vi "disableMenueItem.vi"(3 "error in":errorcluster, 4 "ItemTag":string, 5 "All Devices (h)":string[](array[string]), 6 "MenuRef":refnum<k9>) -> (0 "error out":errorcluster, 1 "this is a Device(tag)":bool, 2 "menu reference out":refnum<k9>)   [LabVIEW 2013]
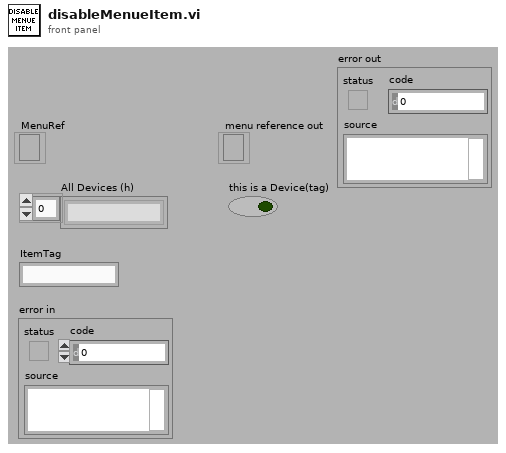
[diagram p1: front panel]
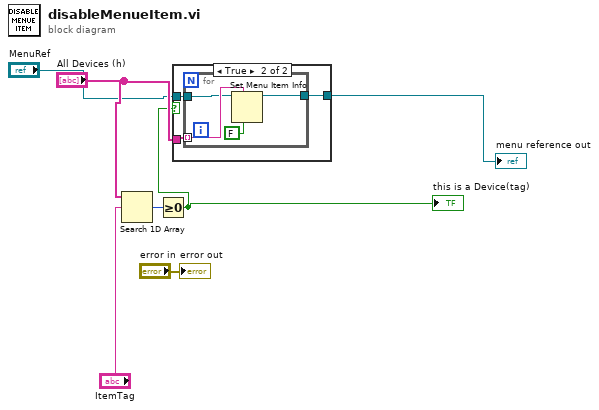
[diagram p0: block diagram]
diagram:
  n1 = Search 1D Array(1D array="All Devices (h)", element="ItemTag") -> (index of element=w3:i32)  [unwired: 1 in]
  n2 = Greater Or Equal To 0?(x=w3) -> (x >= 0?=w5:bool)
  "this is a Device(tag)" <- w5
  n3 = case shown="True" w5 {
    tunnel: "All Devices (h)" -> [_ w11]
    tunnel: "MenuRef" -> [w8 w10]
    tunnel: [w8 w9] -> w6
    frame False {
    }
    frame True {
      n4 = for {
        tunnel: w11 -> [w15] mode=indexing
        tunnel: w10 -> [w13]
        tunnel: [w12] -> w9
        n5 = Set Menu Item Info(6:FALSE ("checked"), 7:w15, 11:w13) -> (3:w12:refnum<k9>)  [unwired: 4 in, 1 out]
      }
    }
  }
  "menu reference out" <- w6
  "error out" <- "error in"
